vi "Process.vi"(8 "error in":errorcluster, 11 "DAQmx":refnum<class "DAQmx.lvclass">) -> (0 "error out":errorcluster, 3 "DAQmx out":refnum<class "DAQmx.lvclass">)   [LabVIEW 2016, in "DAQmx.lvclass"]
doc: "---------------------------------------------------------------\nJKI State Machine Objects™\nhttp://jki.net/state-machine-objects/\nCopyright (C) 2005-2015, JKI <info@jki.net>\nALL RIGHTS RESERVED"
uses:
  DAQmx.lvclass
  C:/Program Files (x86)/National Instruments/LabVIEW 2016/vi.lib/JKI/JKI SMO/SMO/SMO.lvclass
  <vilib>/JKI/JKI SMO/SMO/Typedefs/Parent Call--Enum.ctl
  DAQ/DAQ.lvclass
  <vilib>/JKI/JKI SMO/SMO/SMO.lvclass
panel:
  # "For instructions on how to use the JKI State Machine Objects, examples and video tutorials, visit:\nhttp://jki.net/state-machine-objects/\n\nJKI State Machine Objects™\nhttp://jki.net/state-machine-objects/\nCopyright (C) 2005-2015, JKI <info@jki.net>\nALL RIGHTS RESERVED"
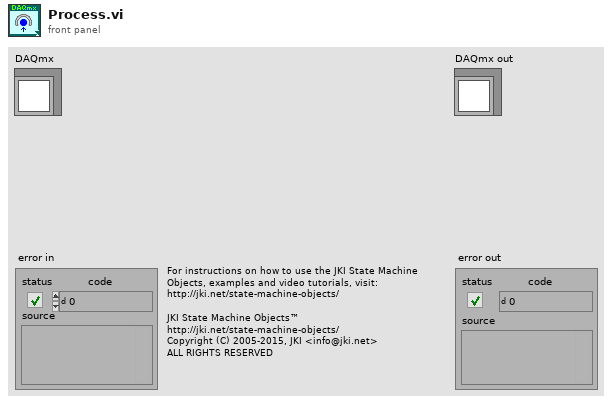
[diagram p1: front panel]
types:
  T1 = typedef "SMO.lvclass/Parent Call--Enum.ctl" = enum16{"Allows parent to run", "Does not request parent to run"}
  T2 = enum32{"invalid app kind", "Development System", "Run Time System", "Student Edition", "Embedded LabVIEW", "Evaluation", "Custom"}
  T3 = enum32{"Invalid", "Standard", "Closed", "Hidden", "Minimized", "Maximized"}
  T4 = enum32{"Bad", "Idle", "Run top level", "Running"}
  T5 = cluster{"Core":cluster{"Current VI Reference":refnum<vi>, "Close Panel on Exit?":bool, "error":errorcluster}, "Self Reference":refnum<class "DAQmx.lvclass">, "Your string data":string}
  T6 = cluster{"Current VI Reference":refnum<vi>, "Close Panel on Exit?":bool, "error":errorcluster}
  T7 = typedef "SMO.lvclass/Protected Events.ctl" = cluster{"StopProcesses":refnum<user-event>, "AbortProcesses":refnum<user-event>, "Config Changed":refnum<user-event>, "Dependency":refnum<user-event>}
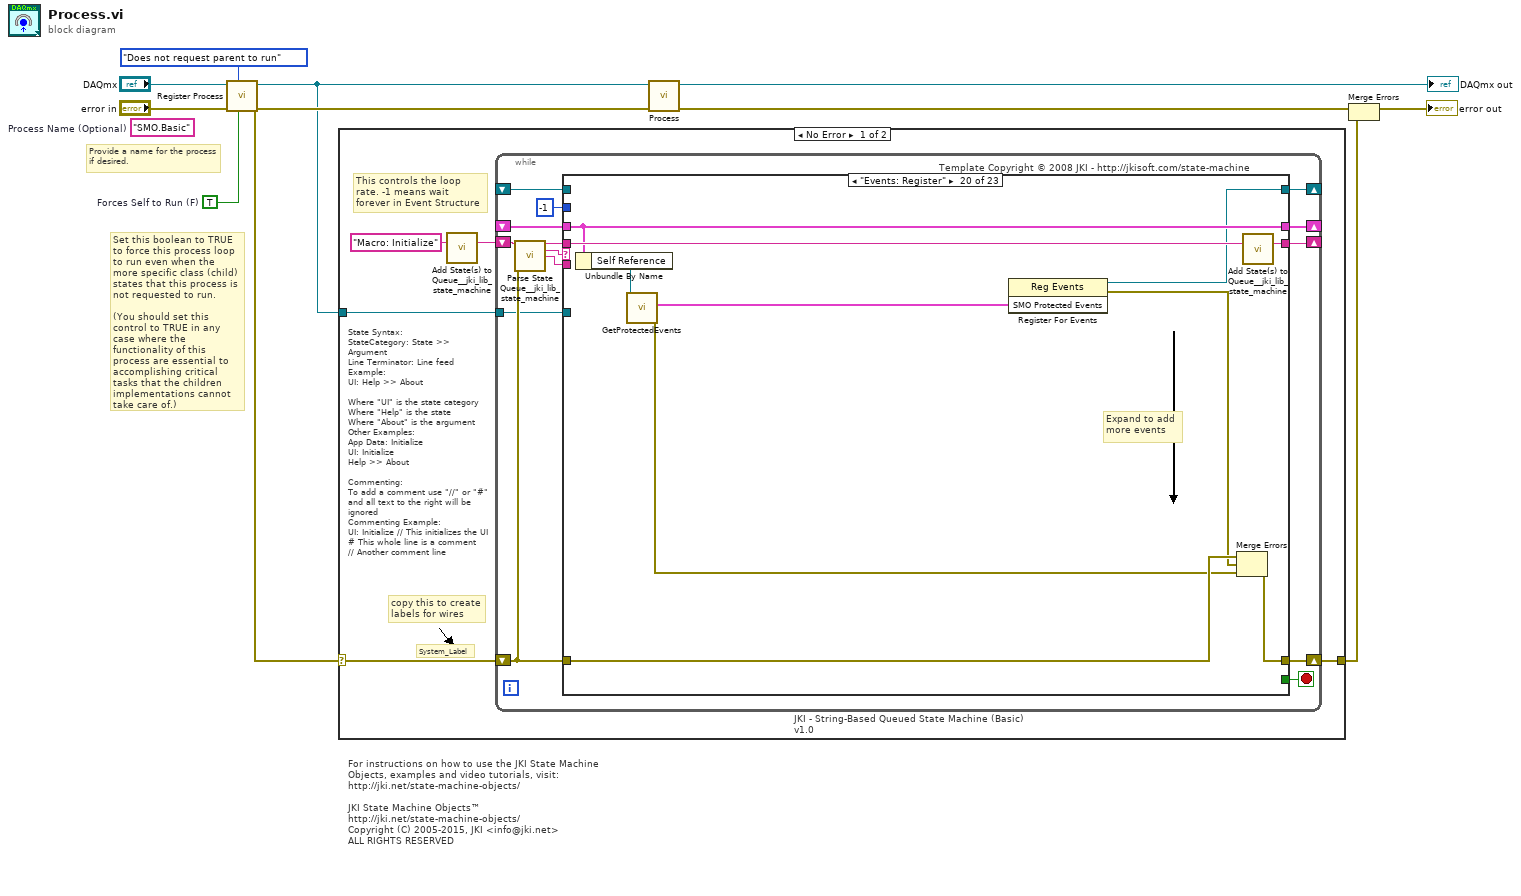
[diagram p0: block diagram]
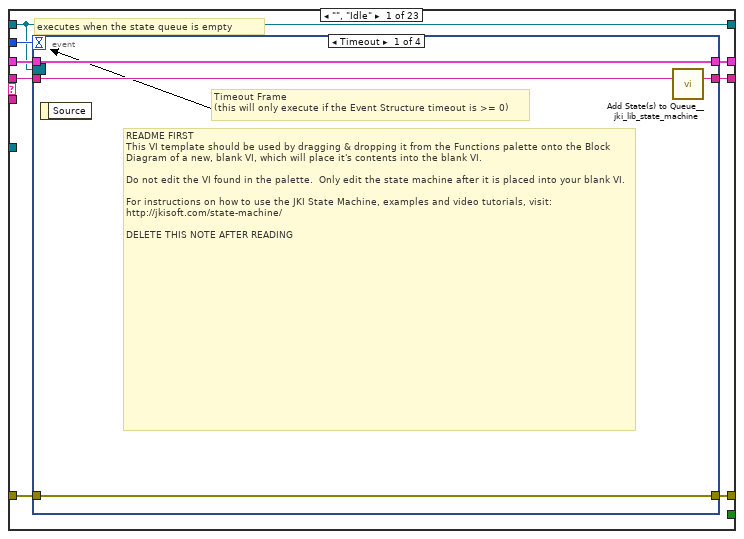
[diagram p2: hidden frame]
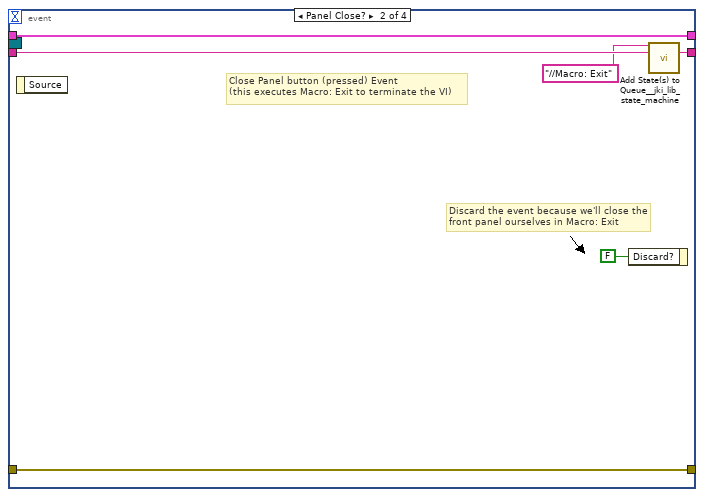
[diagram p3: hidden frame]
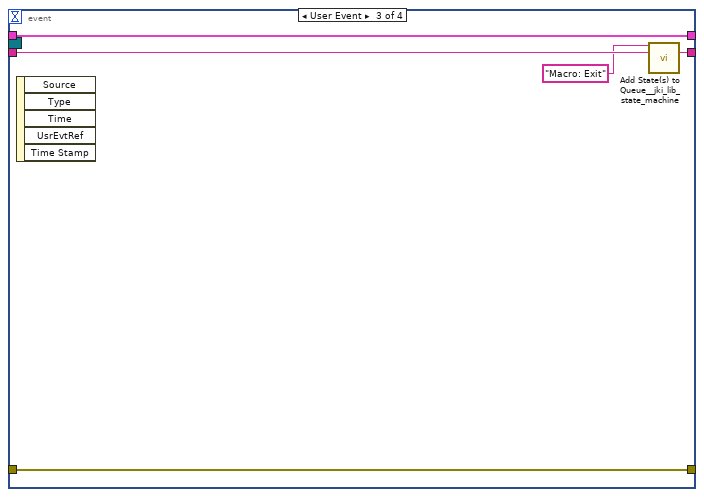
[diagram p4: hidden frame]
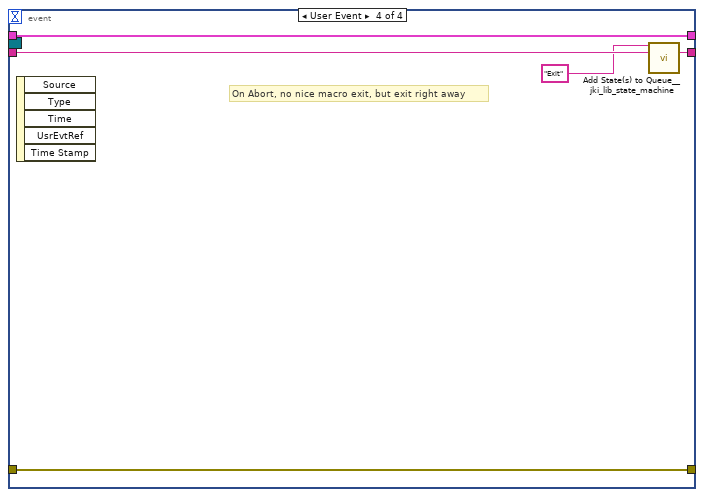
[diagram p5: hidden frame]
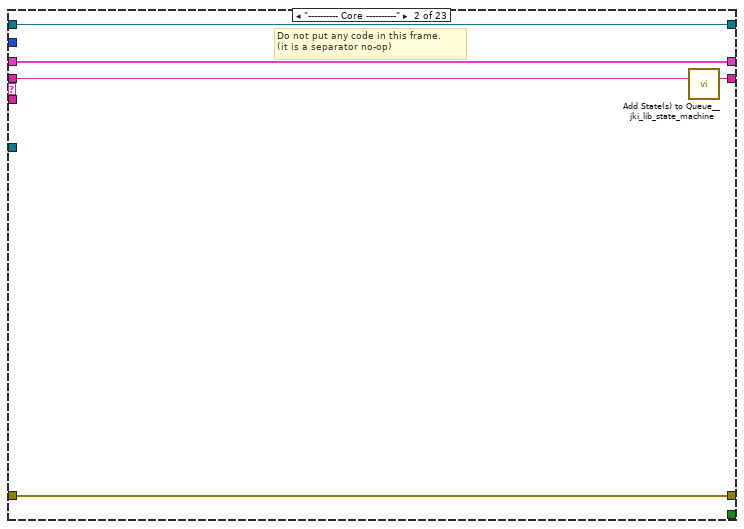
[diagram p6: hidden frame]
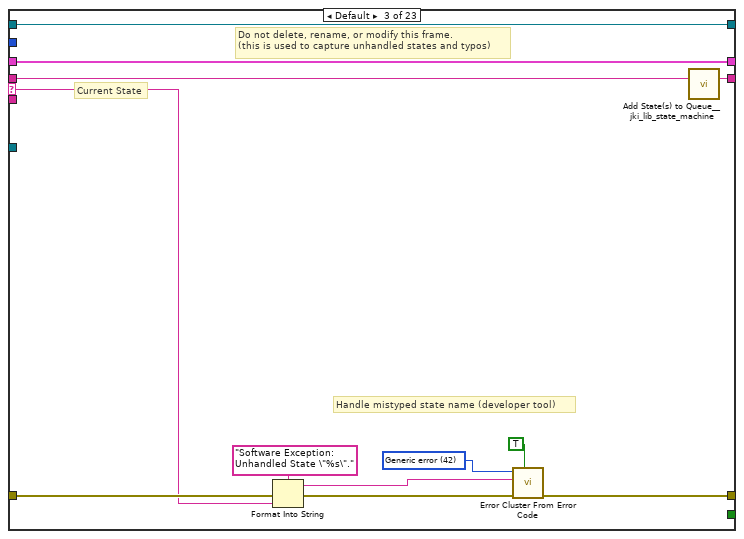
[diagram p7: hidden frame]
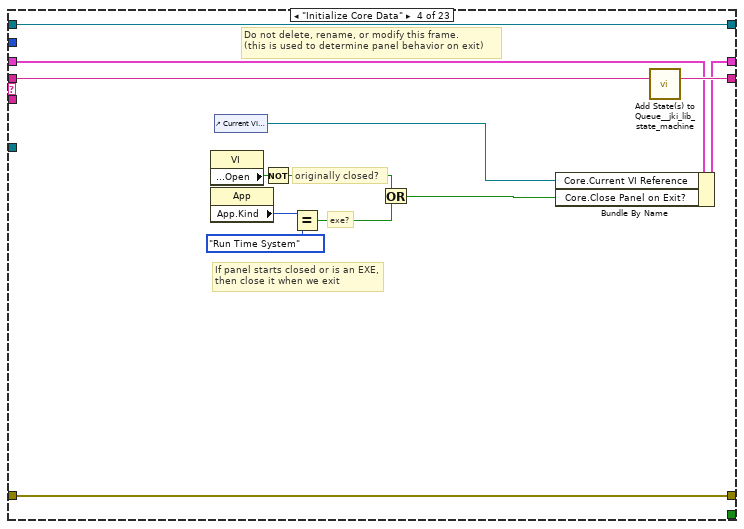
[diagram p8: hidden frame]
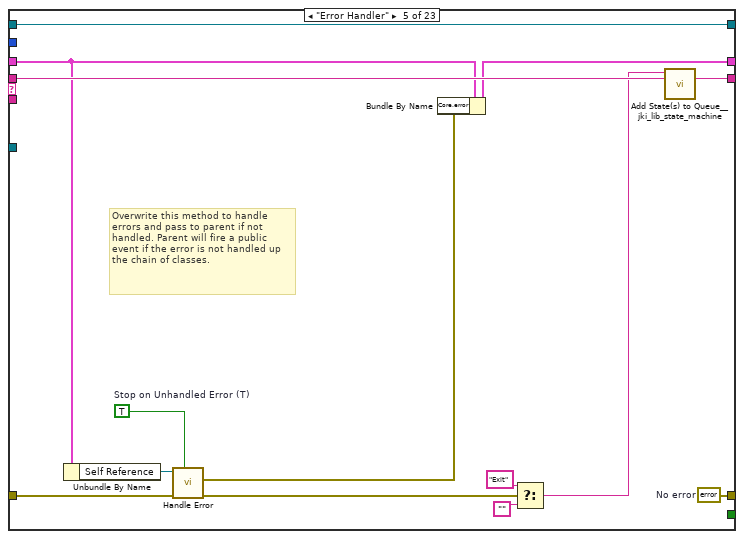
[diagram p9: hidden frame]
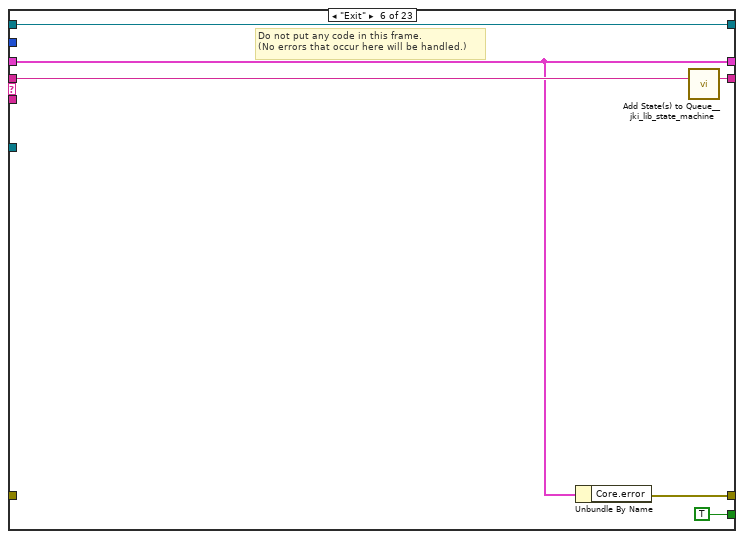
[diagram p10: hidden frame]
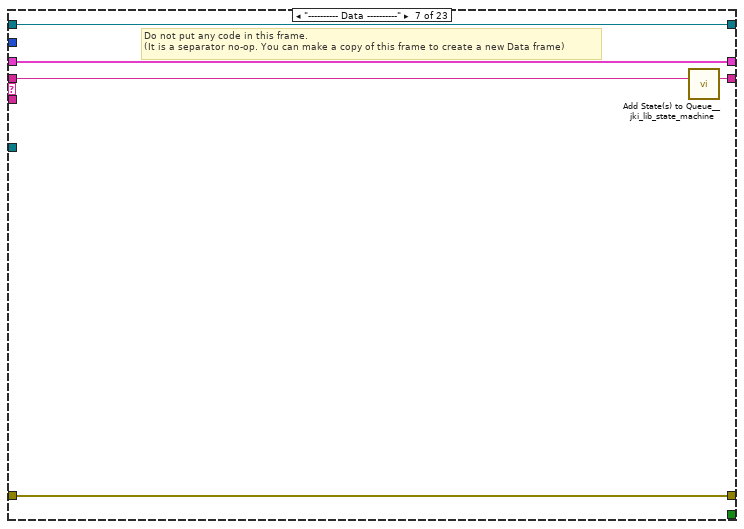
[diagram p11: hidden frame]
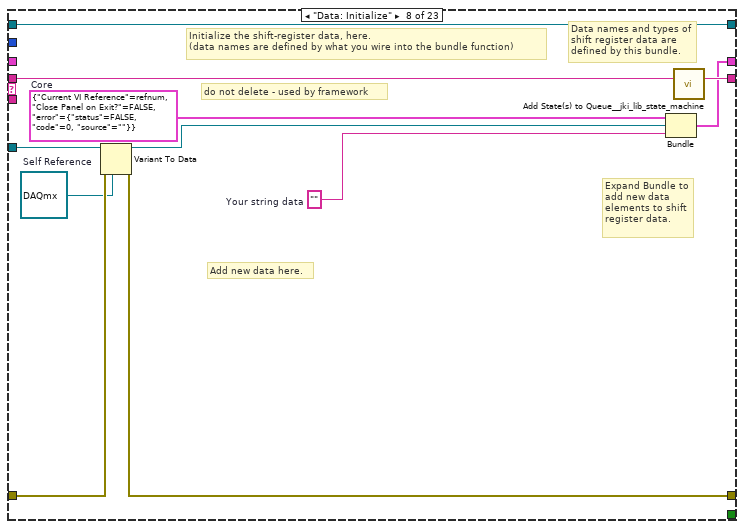
[diagram p12: hidden frame]
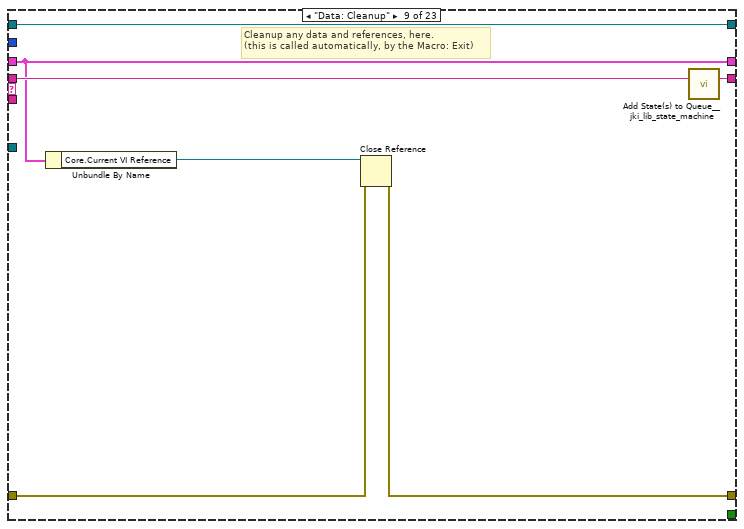
[diagram p13: hidden frame]
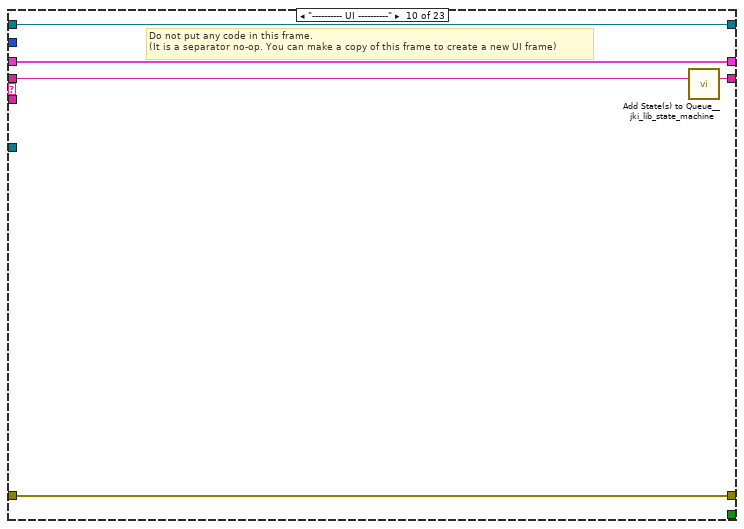
[diagram p14: hidden frame]
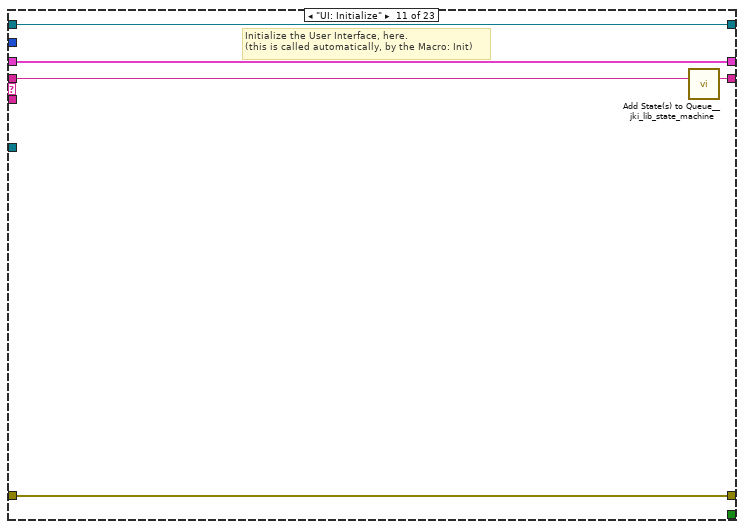
[diagram p15: hidden frame]
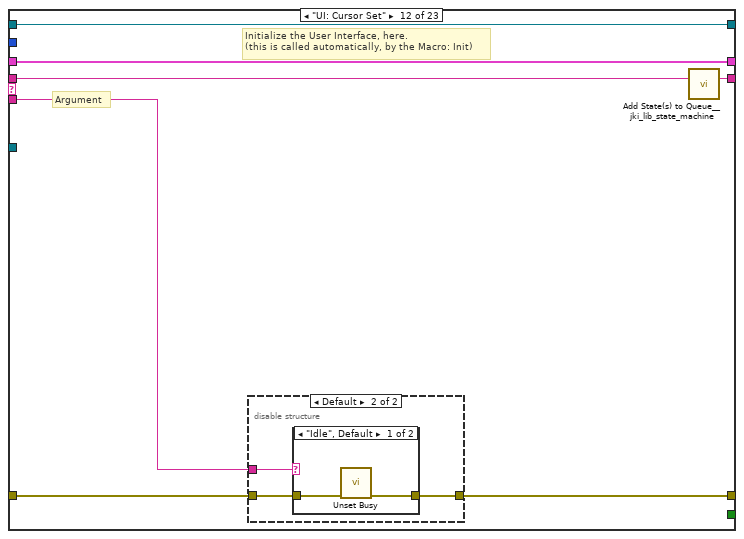
[diagram p16: hidden frame]
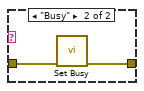
[diagram p18: hidden frame]
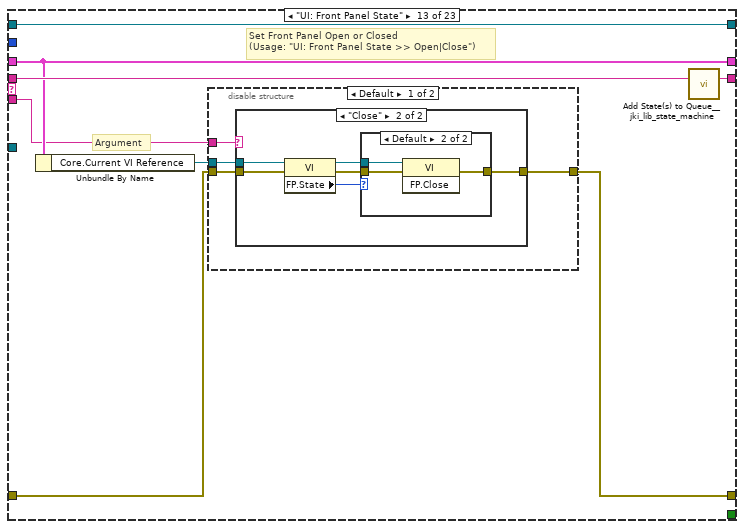
[diagram p19: hidden frame]
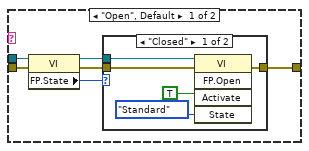
[diagram p20: hidden frame]
diagram:
  w1 = TRUE  # Forces Self to Run (F)
  (unwired) "SMO.Basic"  # Process Name (Optional)
  # "Provide a name for the process\nif desired."
  # "Set this boolean to TRUE to force this process loop to run even when the more specific class (child) states that this process is not requested to run.\n\n(You should set this control to TRUE in any case where the functionality of this process are essential to accomplishing critical tasks that the children implementations cannot take care of.)"
  # "For instructions on how to use the JKI State Machine Objects, examples and video tutorials, visit:\nhttp://jki.net/state-machine-objects/\n\nJKI State Machine Objects™\nhttp://jki.net/state-machine-objects/\nCopyright (C) 2005-2015, JKI <info@jki.net>\nALL RIGHTS RESERVED"
  n1 = call <vilib>:"Register Process.vi"("Forces Self to Run (F)"=w1, "Parent Call"=Parent_Call--Enum."Does not request parent to run", "error in (no error)"="error in", "SMO"="DAQmx") -> ("error out"=w7:errorcluster, "SMO out"=w6:refnum<class "DAQmx.lvclass">)  [unwired: 6 in]
  n2 = case shown="No Error" w7 {
    selector: w7 -> [w12 w273]
    tunnel: w6 -> [w13 _]
    tunnel: [w11 w273] -> w3
    frame No Error {
      # "State Syntax:\nStateCategory: State >> Argument\nLine Terminator: Line feed\nExample:\nUI: Help >> About\n\nWhere \"UI\" is the state category\nWhere \"Help\" is the state\nWhere \"About\" is the argument\nOther Examples:\nApp Data: Initialize\nUI: Initialize\nHelp >> About\n\nCommenting:\nTo add a comment use \"//\" or \"#\" and all text to the right will be ignored\nCommenting Example:\nUI: Initialize // This initializes the UI\n# This whole line is a comment\n// Another comment line"
      # "copy this to create labels for wires"
      # "This controls the loop rate. -1 means wait forever in Event Structure"
      # "System_Label"
      n3 = call <vilib>:"Add State(s) to Queue__jki_lib_state_machine.vi"("State(s) in (\"\")"="Macro: Initialize") -> ("States Out"=w15:string)  [unwired: 14 in]
      n4 = while "JKI - String-Based Queued State Machine (Basic) v1.0" {
        shift-right: [w22] -> _
        shift-left: _ -> [w21]
        shift-right: [w25] -> w11
        shift-left: w12 -> [w19]
        shift-right: [w24] -> _
        shift-left: w15 -> [w26]
        tunnel: w13 -> [w18]
        shift-right: [w17] -> _
        shift-left: _ -> [w16]
        stop <- w23 stop-if-true
        # "Template Copyright © 2008 JKI - http://jkisoft.com/state-machine"
        n5 = call <vilib>:"Parse State Queue__jki_lib_state_machine.vi"("State Queue"=w26, "Error In (no error)"=w19) -> ("Remaining States"=w28:string, "Current State"=w29:string, "Arguments"=w27:string)  [unwired: 11 in]
        n6 = case shown="\"Events: Register\"" w29 {
          selector: w29 -> [_ _ w64 _ _ _ _ _ _ _ _ _ _ _ _ _ _ _ _ _ _ _ _]
          tunnel: w28 -> [w37 w62 w68 w87 w101 w107 w112 w123 w130 w135 w140 w147 w163 w195 w209 w223 w228 w239 w244 w254 w260 w265 w272]
          tunnel: w27 -> [_ _ _ _ _ _ _ _ _ _ _ w141 w157 _ _ _ _ _ _ _ _ _ _]
          tunnel: w21 -> [w35 w59 w66 w78 w95 w103 w109 _ w125 w132 w138 w145 w159 w192 w205 w214 w225 w236 w241 w252 w258 w263 w268]
          tunnel: [w34 w60 w70 w84 w96 w102 w110 w118 w126 w133 w137 w142 w160 w193 w207 w221 w226 w230 w242 w247 w256 w261 w269] -> w25
          tunnel: w19 -> [w33 w60 w69 w84 w97 _ w110 w119 w127 w133 w137 w143 w161 w193 w207 w221 w226 w231 w242 w248 w256 w261 w269]
          tunnel: [w36 w61 w67 w86 w100 w106 w111 w122 w129 w134 w139 w146 w162 w194 w208 w222 w227 w238 w243 w253 w259 w264 w271] -> w24
          tunnel: [_ _ _ _ _ TRUE _ _ _ _ _ _ _ _ _ _ _ _ _ _ _ _ _] -> w23
          tunnel: [w32 w59 w66 w85 w94 w103 w109 w121 w125 w132 w138 w145 w159 w192 w205 w214 w225 w236 w241 w252 w258 w263 w267] -> w22
          tunnel: -1 ("Timeout") -> [w31 _ _ _ _ _ _ _ _ _ _ _ _ _ _ _ _ _ _ _ _ _ _]
          tunnel: w18 -> [_ _ _ _ _ _ _ w116 _ _ _ _ _ _ _ _ _ _ _ _ _ _ _]
          tunnel: [w30 w58 w63 w75 w99 w104 w108 w114 w124 w131 w136 w144 w156 w191 w206 w215 w224 w237 w240 w251 w257 w262 w270] -> w17
          tunnel: w16 -> [w30 w58 w63 w75 w99 w104 w108 w114 w124 w131 w136 w144 w156 w191 w206 w215 w224 w237 w240 _ w257 w262 w270]
          frame "", "Idle" {
            # "executes when the state queue is empty"
            n7 = event shown="[0] Timeout" {
              selector: w30 -> [_ _ _ _]
              dyn-events: _ -> [_ _ _ _]
              timeout: w31 -> [_ _ _ _]
              tunnel: w37 -> [w41 w47 w52 w57]
              tunnel: [w40 w46 w51 w56] -> w36
              tunnel: w35 -> [w39 w44 w49 w54]
              tunnel: [w38 w45 w50 w55] -> w34
              tunnel: w33 -> [w38 w45 w50 w55]
              tunnel: [w39 w44 w49 w54] -> w32
              event Timeout {
                # "README FIRST\nThis VI template should be used by dragging & dropping it from the Functions palette onto the Block Diagram of a new, blank VI, which will place it's contents into the blank VI.\n\nDo not edit the VI found in the palette.  Only edit the state machine after it is placed into your blank VI.\n\nFor instructions on how to use the JKI State Machine, examples and video tutorials, visit:\nhttp://jkisoft.com/state-machine/\n\nDELETE THIS NOTE AFTER READING"
                # "Timeout Frame\n(this will only execute if the Event Structure timeout is >= 0)"
                n8 = event-data() -> ()  [unwired: 1 in, 1 out]
                n9 = call <vilib>:"Add State(s) to Queue__jki_lib_state_machine.vi"("State(s) in (\"\")"=w41) -> ("States Out"=w40:string)  [unwired: 14 in]
              }
              event Panel Close? {
                # "Discard the event because we'll close the front panel ourselves in Macro: Exit"
                # "Close Panel button (pressed) Event\n(this executes Macro: Exit to terminate the VI)"
                n10 = event-data() -> ()  [unwired: 1 in, 1 out]
                n11 = event-data("Discard?"=FALSE) -> ()  [unwired: 1 in, 1 out]
                n12 = call <vilib>:"Add State(s) to Queue__jki_lib_state_machine.vi"("State(s) in Front (\"\")"="//Macro: Exit", "State(s) in (\"\")"=w47) -> ("States Out"=w46:string)  [unwired: 13 in]
              }
              event User Event {
                n13 = event-data() -> ()  [unwired: 1 in, 5 out]
                n14 = call <vilib>:"Add State(s) to Queue__jki_lib_state_machine.vi"("State(s) in Front (\"\")"="Macro: Exit", "State(s) in (\"\")"=w52) -> ("States Out"=w51:string)  [unwired: 13 in]
              }
              event User Event {
                # "On Abort, no nice macro exit, but exit right away"
                n15 = event-data() -> ()  [unwired: 1 in, 5 out]
                n16 = call <vilib>:"Add State(s) to Queue__jki_lib_state_machine.vi"("State(s) in Front (\"\")"="Exit", "State(s) in (\"\")"=w57) -> ("States Out"=w56:string)  [unwired: 13 in]
              }
            }
          }
          frame "---------- Core ----------" {
            # "Do not put any code in this frame.\n(it is a separator no-op)"
            n17 = call <vilib>:"Add State(s) to Queue__jki_lib_state_machine.vi"("State(s) in (\"\")"=w62) -> ("States Out"=w61:string)  [unwired: 14 in]
          }
          frame Default {
            w73 = 42 items=["No error", "Argument error", "Memory is full", "Out of zone", "End of file", "File already open", "Generic file I/O error", "File not found", "File permission error", "Disk is full", "Duplicate path", "Too many files open", "System feature not enabled", "Resource file not found", "Cannot add resource", "Resource not found", "Image not found", "Image memory error", "Pen does not exist", "Config type invalid", "Config token not found", "Config parse error", "Config memory error", "Bad external code format", "Bad external code offset", "External code not present", "Null window", "Destroy window error", "Null menu", "Print aborted", "Bad print record", "Print driver error", "Windows error during printing", "Memory error during printing", "Print dialog error", "Generic print error", "Invalid device refnum", "Device not found", "Device parameter error", "Device unit error", "Cannot open device", "Device call aborted", "Generic error", "Cancelled by user", "Object ID too low", "Object ID too high", "Object not in heap", "Unknown heap", "Unknown object (invalid DefProc)", "Unknown object (DefProc not in table)", "Message out of range", "Invalid (null) method", "Unknown message", "Manager call not supported", "Bad address", "Network operation in progress", "Network operation timed out", "Connection is busy", "Network attribute not supported", "Network error", "Address in use", "System out of memory", "Connection aborted", "Connection refused", "Not connected", "Already connected", "Connection closed", "Initialization error (interapplication manager)", "Bad occurrence", "Wait on unbound occurrence handler", "Occurrence queue overflow", "Datalog type conflict", "Unused", "Unrecognized type (interapplication manager)", "Memory corrupt", "Failed to make temporary DLL", "Old CIN version", "Drag socket not found", "Failed to load drop-object", "Failed to register OLE object", "Failed to release OLE object", "Format specifier type mismatch", "Unknown format specifier", "Too few format specifiers", "Too many format specifiers", "Scan failed", "Newer CIN version", "Error converting to variant", "Runtime menu error", "Password tampered", "Variant attribute not found", "Incompatible variant data type", "Event data is not available", "Event Store is not present", "Occurrence is not found", "Event Queue is not created", "Event info is not available", "Refnum passed is NULL", "Error retrieving Class GUID", "Error retrieving CoClass GUID", "Error retrieving TypeLib GUID.", "Bad built application magic bytes.", "Specific driver is different from the specific driver associated with the Logical Name.", "There is no session opened to the class driver.", "Max Error", "MAX - Error with config objects", "MAX - Error loading configuration", "MAX - Group not supported"]
            # "Current State"
            # "Do not delete, rename, or modify this frame.\n(this is used to capture unhandled states and typos)"
            # "Handle mistyped state name (developer tool)"
            n18 = Format Into String(format string="Software Exception: Unhandled State \"%s\"." ("message"), error in=w69, w64) -> (resulting string=w72:string, error out=w71:errorcluster)  [unwired: 1 in]
            n19 = call <vilib>:"Error Cluster From Error Code.vi"("show call chain? (False)"=TRUE, "error in (no error)"=w71, "error message (\"\")"=w72, "error code (0)"=w73) -> ("error out"=w70:errorcluster)  [unwired: 5 in]
            n20 = call <vilib>:"Add State(s) to Queue__jki_lib_state_machine.vi"("State(s) in (\"\")"=w68) -> ("States Out"=w67:string)  [unwired: 14 in]
          }
          frame "Initialize Core Data" {
            # "Do not delete, rename, or modify this frame.\n(this is used to determine panel behavior on exit)"
            # "originally closed?"
            # "exe?"
            # "If panel starts closed or is an EXE, then close it when we exit"
            n21 = property class="VI"() -> ("Front Panel.Open"=w83:bool)  [unwired: 2 in, 2 out]
            n22 = property class="App"() -> ("App.Kind"=w82:T2)  [unwired: 2 in, 2 out]
            n23 = control-ref of="Current VI Reference"() -> (w76:refnum<vi>)
            n24 = Not(x=w83) -> (.not. x?=w80:bool)
            n25 = Equal?(x=w82, y=T2."Run Time System" ("Application:Kind")) -> (x = y?=w79:bool)
            n26 = Or(x=w80, y=w79) -> (x .or. y?=w77:bool)
            n27 = Bundle By Name(cluster=w78, "Core.Current VI Reference"=w76, "Core.Close Panel on Exit?"=w77) -> (w85:T5)
            n28 = call <vilib>:"Add State(s) to Queue__jki_lib_state_machine.vi"("State(s) in (\"\")"=w87) -> ("States Out"=w86:string)  [unwired: 14 in]
          }
          frame "Error Handler" {
            w88 = TRUE  # Stop on Unhandled Error (T)
            w96 = errorcluster {"status"=FALSE, "code"=0, "source"=""}  # No error
            # "Overwrite this method to handle errors and pass to parent if not handled. Parent will fire a public event if the error is not handled up the chain of classes."
            n29 = Unbundle By Name(w95) -> ("Self Reference"=w98:refnum<class "DAQmx.lvclass">)
            n30 = call-dynamic "Handle Error.vi"("Stop on Unhandled Error (T)"=w88, "error in"=w97, "SMO"=w98) -> ("handling error"=w89:errorcluster, "Unhandled error"=w92:errorcluster)  [unwired: 6 in, 1 out]
            n31 = Bundle By Name(cluster=w95, "Core.error"=w92) -> (w94:T5)
            n32 = Select(t="Exit", s=w89, f="") -> (s? t:f=w93:string)
            n33 = call <vilib>:"Add State(s) to Queue__jki_lib_state_machine.vi"("State(s) in Front (\"\")"=w93, "State(s) in (\"\")"=w101) -> ("States Out"=w100:string)  [unwired: 13 in]
          }
          frame "Exit" {
            # "Do not put any code in this frame.\n(No errors that occur here will be handled.)"
            n34 = Unbundle By Name(w103) -> ("Core.error"=w102:errorcluster)
            n35 = call <vilib>:"Add State(s) to Queue__jki_lib_state_machine.vi"("State(s) in (\"\")"=w107) -> ("States Out"=w106:string)  [unwired: 14 in]
          }
          frame "---------- Data ----------" {
            # "Do not put any code in this frame.\n(It is a separator no-op. You can make a copy of this frame to create a new Data frame)"
            n36 = call <vilib>:"Add State(s) to Queue__jki_lib_state_machine.vi"("State(s) in (\"\")"=w112) -> ("States Out"=w111:string)  [unwired: 14 in]
          }
          frame "Data: Initialize" {
            w113 = T6 {"Current VI Reference"=refnum, "Close Panel on Exit?"=FALSE, "error"={"status"=FALSE, "code"=0, "source"=""}}  # Core
            w117 = refnum<class "DAQmx.lvclass"> refnum  # Self Reference
            w120 = ""  # Your string data
            # "do not delete - used by framework"
            # "Expand Bundle to add new data elements to shift register data."
            # "Add new data here."
            # "Data names and types of shift register data are defined by this bundle."
            # "Initialize the shift-register data, here.\n(data names are defined by what you wire into the bundle function)"
            n37 = Variant To Data(error in=w119, type=w117, Variant=w116) -> (data=w115:refnum<class "DAQmx.lvclass">, error out=w118:errorcluster)
            n38 = Bundle("Core"=w113, "Self Reference"=w115, "Your string data"=w120) -> (w121:T5)  [unwired: 1 in]
            n39 = call <vilib>:"Add State(s) to Queue__jki_lib_state_machine.vi"("State(s) in (\"\")"=w123) -> ("States Out"=w122:string)  [unwired: 14 in]
          }
          frame "Data: Cleanup" {
            # "Cleanup any data and references, here.\n(this is called automatically, by the Macro: Exit)"
            n40 = Unbundle By Name(w125) -> ("Core.Current VI Reference"=w128:refnum<vi>)
            n41 = Close Reference(reference=w128, error in (no error)=w127) -> (error out=w126:errorcluster)
            n42 = call <vilib>:"Add State(s) to Queue__jki_lib_state_machine.vi"("State(s) in (\"\")"=w130) -> ("States Out"=w129:string)  [unwired: 14 in]
          }
          frame "---------- UI ----------" {
            # "Do not put any code in this frame.\n(It is a separator no-op. You can make a copy of this frame to create a new UI frame)"
            n43 = call <vilib>:"Add State(s) to Queue__jki_lib_state_machine.vi"("State(s) in (\"\")"=w135) -> ("States Out"=w134:string)  [unwired: 14 in]
          }
          frame "UI: Initialize" {
            # "Initialize the User Interface, here.\n(this is called automatically, by the Macro: Init)"
            n44 = call <vilib>:"Add State(s) to Queue__jki_lib_state_machine.vi"("State(s) in (\"\")"=w140) -> ("States Out"=w139:string)  [unwired: 14 in]
          }
          frame "UI: Cursor Set" {
            # "Argument"
            # "Initialize the User Interface, here.\n(this is called automatically, by the Macro: Init)"
            n45 = disable-structure shown="Default" {
              disable-tunnel: w143 -> [w148 w151]
              disable-tunnel: [w148 w150] -> w142
              disable-tunnel: w141 -> [_ w149]
              frame condition #0 {
              }
              frame condition #1 (active) {
                n46 = case shown="\"Idle\", Default" w149 {
                  tunnel: w151 -> [w153 w155]
                  tunnel: [w152 w154] -> w150
                  frame "Idle", Default {
                    n47 = call <vilib>:"Unset Busy.vi"("error in (no error)"=w153) -> ("error out"=w152:errorcluster)  [unwired: 10 in]
                  }
                  frame "Busy" {
                    n48 = call <vilib>:"Set Busy.vi"("error in (no error)"=w155) -> ("error out"=w154:errorcluster)  [unwired: 9 in, 1 out]
                  }
                }
              }
            }
            n49 = call <vilib>:"Add State(s) to Queue__jki_lib_state_machine.vi"("State(s) in (\"\")"=w147) -> ("States Out"=w146:string)  [unwired: 14 in]
          }
          frame "UI: Front Panel State" {
            # "Argument"
            # "Set Front Panel Open or Closed\n(Usage: \"UI: Front Panel State >> Open|Close\")"
            n50 = Unbundle By Name(w159) -> ("Core.Current VI Reference"=w158:refnum<vi>)
            n51 = disable-structure shown="Default" {
              disable-tunnel: w161 -> [w167 w190]
              disable-tunnel: [w166 w190] -> w160
              disable-tunnel: w158 -> [w165 _]
              disable-tunnel: w157 -> [w164 _]
              frame condition #0 (active) {
                n52 = case shown="\"Close\"" w164 {
                  tunnel: w167 -> [w171 w184]
                  tunnel: [w173 w185] -> w166
                  tunnel: w165 -> [w172 w182]
                  frame "Open", Default {
                    n53 = property class="VI"(reference=w172, error in=w171) -> (reference out=w169:refnum<vi>, error out=w170:errorcluster, "FP.State"=w168:T3)
                    n54 = case shown="\"Closed\"" w168 {
                      tunnel: [w176 w179] -> w173
                      tunnel: w170 -> [w175 w179]
                      tunnel: w169 -> [w174 _]
                      frame "Closed" {
                        n55 = invoke class="VI" method="FP.Open"(reference=w174, error in=w175, "Activate"=TRUE, "State"=T3."Standard") -> (error out=w176:errorcluster)  [unwired: 1 in, 4 out]
                      }
                      frame Default {
                      }
                    }
                  }
                  frame "Close" {
                    n56 = property class="VI"(reference=w182, error in=w184) -> (reference out=w181:refnum<vi>, error out=w183:errorcluster, "FP.State"=w180:T3)
                    n57 = case shown="Default" w180 {
                      tunnel: [w186 w189] -> w185
                      tunnel: w183 -> [w186 w188]
                      tunnel: w181 -> [_ w187]
                      frame "Invalid", "Closed" {
                      }
                      frame Default {
                        n58 = invoke class="VI" method="FP.Close"(reference=w187, error in=w188) -> (error out=w189:errorcluster)  [unwired: 1 in, 2 out]
                      }
                    }
                  }
                }
              }
              frame condition #1 {
              }
            }
            n59 = call <vilib>:"Add State(s) to Queue__jki_lib_state_machine.vi"("State(s) in (\"\")"=w163) -> ("States Out"=w162:string)  [unwired: 14 in]
          }
          frame "---------- Macro ----------" {
            # "Do not put any code in this frame.\n(It is a separator no-op. You can make a copy of this frame to create a new Macro frame)"
            n60 = call <vilib>:"Add State(s) to Queue__jki_lib_state_machine.vi"("State(s) in (\"\")"=w195) -> ("States Out"=w194:string)  [unwired: 14 in]
          }
          frame "Macro: Initialize" {
            w200 = "//UI: Initialize\n//UI: Front Panel State >> Open"  # //UI: Initialize //UI: Front Panel State >> Open
            w196 = "Process: Sync"
            # "Initialization Macro\n(This is called once, when the VI starts)"
            n61 = control-ref of="This VI"() -> (w198:refnum<vi>)
            n62 = property class="VI"(reference=w198) -> ("Exec.State"=w197:T4)  [unwired: 1 in, 2 out]
            n63 = Equal?(x=w197, y=T4."Run top level") -> (x = y?=w203:bool)
            n64 = Select(t=w196, s=w203, f="") -> ()  [unwired: 1 out]
            n65 = call <vilib>:"Add State(s) to Queue__jki_lib_state_machine.vi"("State(s) in Front (\"\")"="Data: Initialize\nInitialize Core Data\nEvents: Register", "State(s) in (\"\")"=w196, "State(s) at Back (\"\")"=w200) -> ("States Out"=w199:string)  [unwired: 12 in]
            n66 = call <vilib>:"Add State(s) to Queue__jki_lib_state_machine.vi"("State(s) in Front (\"\")"=w199, "State(s) in (\"\")"=w209) -> ("States Out"=w208:string)  [unwired: 13 in]
          }
          frame "Macro: Exit" {
            # "Exit Macro\n(This is called once, when the VI exits)"
            n67 = Unbundle By Name(w214) -> ("Core.Close Panel on Exit?"=w220:bool)
            n68 = Select(t="UI: Front Panel State >> Close", s=w220, f="") -> (s? t:f=w217:string)
            n69 = call <vilib>:"Add State(s) to Queue__jki_lib_state_machine.vi"("State(s) in Front (\"\")"="Data: Cleanup\nEvents: Unregister", "State(s) in (\"\")"="Process: Sync", "State(s) at Back (\"\")"="Exit") -> ("States Out"=w211:string)  [unwired: 12 in]
            n70 = call <vilib>:"Add State(s) to Queue__jki_lib_state_machine.vi"("State(s) in (\"\")"=w217, "State(s) at Back (\"\")"=w211) -> ("States Out"=w216:string)  [unwired: 13 in]
            n71 = call <vilib>:"Add State(s) to Queue__jki_lib_state_machine.vi"("State(s) in Front (\"\")"=w216, "State(s) in (\"\")"=w223) -> ("States Out"=w222:string)  [unwired: 13 in]
          }
          frame "---------- Process ----------" {
            # "Template Separator\n(You can make a copy of, or modify, this frame)"
            n72 = call <vilib>:"Add State(s) to Queue__jki_lib_state_machine.vi"("State(s) in (\"\")"=w228) -> ("States Out"=w227:string)  [unwired: 14 in]
          }
          frame "Process: Sync" {
            n73 = Unbundle By Name(w236) -> ("Self Reference"=w232:refnum<class "DAQmx.lvclass">)
            n74 = call <vilib>:"WaitOnProcessSync.vi"("error in (no error)"=w231, "SMO"=w232) -> ("error out"=w230:errorcluster, "Don't run?"=w235:bool)  [unwired: 7 in, 1 out]
            n75 = Select(t="Data: Cleanup\nEvents: Unregister\nExit", s=w235, f="") -> (s? t:f=w229:string)
            n76 = call <vilib>:"Add State(s) to Queue__jki_lib_state_machine.vi"("State(s) in Front (\"\")"=w229, "State(s) in (\"\")"=w239) -> ("States Out"=w238:string)  [unwired: 13 in]
          }
          frame "---------- Events ----------" {
            # "Template Separator\n(You can make a copy of, or modify, this frame)"
            n77 = call <vilib>:"Add State(s) to Queue__jki_lib_state_machine.vi"("State(s) in (\"\")"=w244) -> ("States Out"=w243:string)  [unwired: 14 in]
          }
          frame "Events: Register" {
            # "Expand to add\nmore events"
            n78 = Unbundle By Name(w252) -> ("Self Reference"=w249:refnum<class "DAQmx.lvclass">)
            n79 = call <vilib>:"GetProtectedEvents.vi"("SMO"=w249) -> ("error out"=w245:errorcluster, "SMO Protected Events"=w250:T7)  [unwired: 8 in, 1 out]
            n80 = register-events(w250) -> (reference out=w251:refnum<event-registration>, error out=w246:errorcluster)  [unwired: 2 in]
            n81 = Merge Errors(w248, w246, w245) -> (w247:errorcluster)
            n82 = call <vilib>:"Add State(s) to Queue__jki_lib_state_machine.vi"("State(s) in (\"\")"=w254) -> ("States Out"=w253:string)  [unwired: 14 in]
          }
          frame "Events: Unregister" {
            n83 = Unregister For Events(event registration refnum=w257, error in=w256) -> (error out=w255:errorcluster)
            n84 = call <vilib>:"Clear Errors.vi"("error in (no error)"=w255) -> ()  [unwired: 5 in, 2 out]
            n85 = call <vilib>:"Add State(s) to Queue__jki_lib_state_machine.vi"("State(s) in (\"\")"=w260) -> ("States Out"=w259:string)  [unwired: 14 in]
          }
          frame "---------- Action ----------" {
            n86 = call <vilib>:"Add State(s) to Queue__jki_lib_state_machine.vi"("State(s) in (\"\")"=w265) -> ("States Out"=w264:string)  [unwired: 14 in]
          }
          frame "Action: Template" {
            n87 = Unbundle By Name(w268) -> ("Self Reference"=w266:refnum<class "DAQmx.lvclass">)
            n88 = Bundle By Name(cluster=w268, "Self Reference"=w266) -> (w267:T5)
            n89 = call <vilib>:"Add State(s) to Queue__jki_lib_state_machine.vi"("State(s) in (\"\")"=w272) -> ("States Out"=w271:string)  [unwired: 14 in]
          }
        }
      }
    }
    frame Error {
    }
  }
  n90 = call-parent "Process.vi"("error in"=w7, "DAQ"=w6) -> ("error out"=w4:errorcluster, "DAQ out"=→"DAQmx out":refnum<class "DAQmx.lvclass">)  [unwired: 8 in]
  n91 = Merge Errors(w4, w3) -> (→"error out":errorcluster)
